vi "PowerStatus.vi"(8 "error in (no error)":errorcluster, 11 "DAQmxTaskContainer in":refnum<class "DAQmxTaskContainer.lvclass">) -> (0 "error out":errorcluster, 2 "On/Off":bool, 3 "DAQmxTaskContainer out":refnum<class "DAQmxTaskContainer.lvclass">)   [LabVIEW 2015, in "DAQmxTaskContainer.lvclass"]
uses:
  DAQmxTaskContainer.lvclass
  DAQmxTaskAICurrent.lvclass
  DAQmxTaskAICurrent.lvclass/DAQmxTaskAICurrent.ctl
  DAQmxTaskContainer_General/DAQmxTaksContainer_General.lvclass
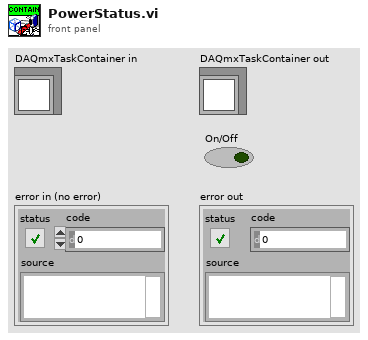
[diagram p1: front panel]
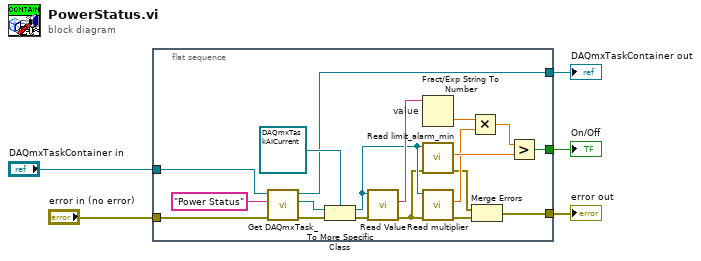
[diagram p0: block diagram]
diagram:
  n1 = flat-sequence {
    tunnel: "error in (no error)" -> [w21]
    tunnel: "DAQmxTaskContainer in" -> [w20]
    tunnel: [w6] -> w4
    tunnel: [w15] -> w3
    tunnel: [w14] -> w5
    frame #0 {
      n2 = call "Get DAQmxTask_.vi"("error in (no error)"=w21, "Task name"="Power Status", "DAQmxTaksContainer_General in"=w20) -> ("error out"=w17:errorcluster, "DAQmx Task"=w18:refnum<class "DAQmxTask.lvclass">, "DAQmxTaksContainer_General out"=w14:refnum<class "DAQmxTaskContainer.lvclass">)  [unwired: 6 in]
      n3 = To More Specific Class(target class=refnum<class "DAQmxTaskAICurrent.lvclass"> refnum ("DAQmxTaskAICurrent.lvclass"), reference=w18, error in=w17) -> (specific class reference=w13:refnum<class "DAQmxTaskAICurrent.lvclass">, error out=w16:errorcluster)
      n4 = call-dynamic "Read Value.vi"("error in (no error)"=w16, "DAQmxTaskAICurrent en entrée"=w13) -> ("error out"=w12:errorcluster, "Data string"=w23:string)  [unwired: 6 in, 2 out]
      n5 = Fract/Exp String To Number "value"(string=w23) -> (number=w11:dbl)  [unwired: 3 in, 1 out]
      n6 = call "Read limit_alarm_min.vi"("error in (no error)"=w12, "DAQmxTaskAICurrent en entrée"=w13) -> ("error out"=w8:errorcluster, "limit_alarm_min"=w24:dbl)  [unwired: 7 in, 1 out]
      n7 = call "Read multiplier.vi"("error in (no error)"=w12, "DAQmxTaskAICurrent en entrée"=w13) -> ("error out"=w7:errorcluster, "multiplier"=w10:dbl)  [unwired: 7 in, 1 out]
      n8 = Multiply(x=w11, y=w10) -> (x*y=w9:dbl)
      n9 = Merge Errors(w8, w7) -> (w6:errorcluster)
      n10 = Greater?(x=w9, y=w24) -> (0:w15:bool)
    }
  }
  "DAQmxTaskContainer out" <- w5
  "error out" <- w4
  "On/Off" <- w3
